vi "Initialize.vi"(8 "error in (no error)":errorcluster) -> (0 "error out":errorcluster, 3 "Telegram Class out":refnum<class "Telegram Class.lvclass">)   [LabVIEW 2015, in "Telegram Library.lvlib" / "Telegram Class.lvclass"]
doc: "Created IvanLis by LabVIEW Portal\nProfile: http://labviewportal.org/memberlist.php?mode=viewprofile&u=987\neMail: IvanLisanov@gMail.com\nTelegram: https://t.me/IvanLis"
uses:
  Telegram Class.lvclass
  TypeDef/User.ctl
  TypeDef/Chat.ctl
  TypeDef/Message.ctl
  Telegram Class.lvclass/Telegram Class.ctl
  Telegram Library.lvlib
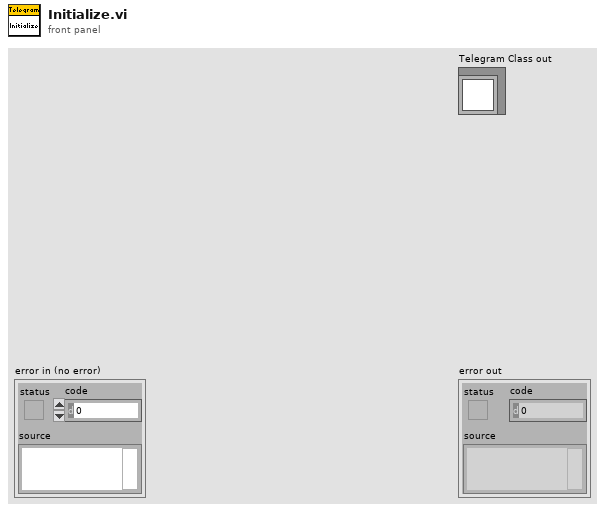
[diagram p1: front panel]
types:
  T1 = typedef "Telegram Library.lvlib/Message.ctl" = cluster{"id":i64, "chat_id":i64, "sender_user_id":i64, "date UTC":timestamp, "content_text":string}
  T2 = typedef "Telegram Library.lvlib/Chat.ctl" = cluster{"id":i64, "position":i64, "title":string}
  T3 = typedef "Telegram Library.lvlib/User.ctl" = cluster{"id":i64, "phone_number":string, "username":string, "last_name":string, "first_name":string}
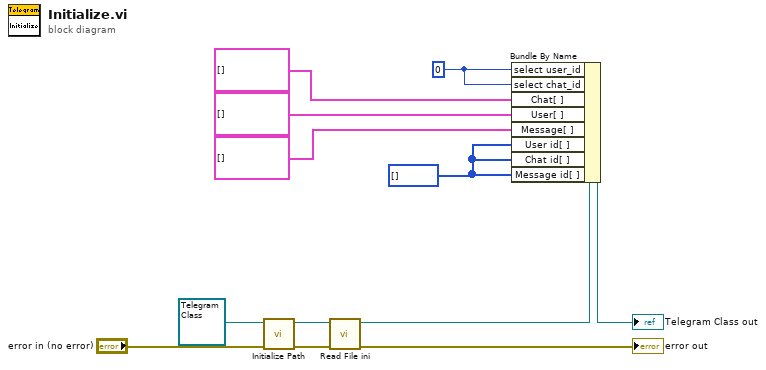
[diagram p0: block diagram]
diagram:
  w2 = i64[] [] ("User id[ ]")
  w5 = i64 0 ("select user_id")
  n1 = call-dynamic "Initialize Path.vi"("error in (no error)"="error in (no error)", "Telegram Class in"=refnum<class "Telegram Class.lvclass"> refnum) -> ("error out"=w10:errorcluster, "Telegram Class out"=w9:refnum<class "Telegram Class.lvclass">)  [unwired: 8 in]
  n2 = call-dynamic "Read File ini.vi"("error in (no error)"=w10, "Telegram Class in"=w9) -> ("error out"=→"error out":errorcluster, "Telegram Class out"=w4:refnum<class "Telegram Class.lvclass">)  [unwired: 8 in]
  n3 = Bundle By Name(cluster=w4, "select user_id"=w5, "select chat_id"=w5, "Chat[ ]"=T2[] [], "User[ ]"=T3[] [], "Message[ ]"=T1[] [], "User id[ ]"=w2, "Chat id[ ]"=w2, "Message id[ ]"=w2) -> (→"Telegram Class out":refnum<class "Telegram Class.lvclass">)
